vi "Channel to Multiplexer.vi"(9 "Polarity (F: Negative, T: Positive)":bool=TRUE, 11 "Multiplexer":T1) -> (1 "ext. Voltmeter":T2=enum."Short AC Sampler", 2 "Nulldetector":T2=enum."Short AC Sampler", 3 "Channel":T2=enum."Short AC Sampler")   [LabVIEW 2019, in "ACSVcontrol-driver.lvlib"]
doc: "Returns setting of multiplexer for selected polarity and channel. Does not set any devices, this is only to simplify setting of multiplexer.\n\nOutput \"Channel\" is used for setup JVS-nulldetector-DUT.\nOutput \"Nulldetector\" is used for direct measurement of DUT using nulldetector.\nOutput \"ext. Voltmeter\" is used for direct measurement of DUT using external voltmeter."
uses:
  ACSVcontrol-driver.lvlib
  Type Definitions/Multiplexer.ctl
  Type Definitions/Measurement Channel.ctl
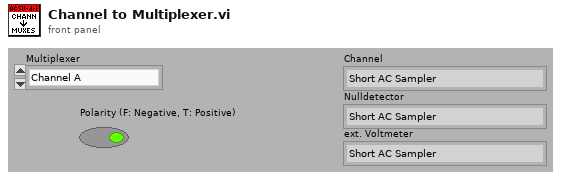
[diagram p1: front panel]
types:
  T1 = typedef "ACSVcontrol-driver.lvlib/Measurement Channel.ctl" = enum16{"Channel A", "Channel B", "Channel C"}
  T2 = typedef "ACSVcontrol-driver.lvlib/Multiplexer.ctl" = enum16{"Short DC Nano / Voltmeter", "Short AC Sampler", "Short Switch DC (JVS->Nano)", "Short Switch AC (JVS->Digit)", "JVS-Voltmeter", "Channel A positive", "Channel A negative", "Channel B positive", "Channel B negative", "Channel C positive", "Channel C negative", "Nulldetector-Channel A+", "Nulldetector-Channel A-", "Nulldetector-Channel B+", "Nulldetector-Channel B-", "Nulldetector-Channel C+", "Nulldetector-Channel C-", "ext.Voltmeter-Channel A+", "ext.Voltmeter-Channel A-", "ext.Voltmeter-Channel B+", "ext.Voltmeter-Channel B-", "ext.Voltmeter-Channel C+", "ext.Voltmeter-Channel C-"}
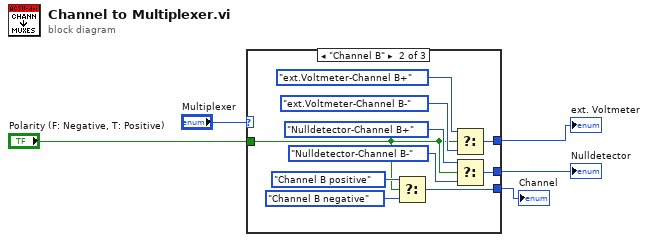
[diagram p0: block diagram]
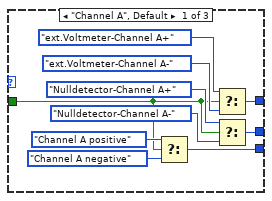
[diagram p2: hidden frame]
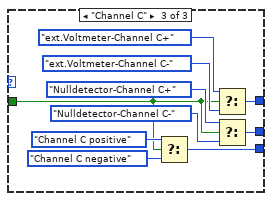
[diagram p3: hidden frame]
diagram:
  n1 = case shown="\"Channel B\"" "Multiplexer" {
    tunnel: "Polarity (F: Negative, T: Positive)" -> [w9 w19 w29]
    tunnel: [w8 w18 w28] -> w4
    tunnel: [w7 w17 w27] -> w3
    tunnel: [w6 w16 w26] -> w2
    frame "Channel A", Default {
      n2 = Select(t=Multiplexer."Channel A positive" ("Multiplexer"), s=w9, f=Multiplexer."Channel A negative" ("Multiplexer")) -> (s? t:f=w8:T2)
      n3 = Select(t=Multiplexer."ext.Voltmeter-Channel A+" ("Multiplexer"), s=w9, f=Multiplexer."ext.Voltmeter-Channel A-" ("Multiplexer")) -> (s? t:f=w6:T2)
      n4 = Select(t=Multiplexer."Nulldetector-Channel A+" ("Multiplexer"), s=w9, f=Multiplexer."Nulldetector-Channel A-" ("Multiplexer")) -> (s? t:f=w7:T2)
    }
    frame "Channel B" {
      n5 = Select(t=Multiplexer."Channel B positive" ("Multiplexer"), s=w19, f=Multiplexer."Channel B negative" ("Multiplexer")) -> (s? t:f=w18:T2)
      n6 = Select(t=Multiplexer."ext.Voltmeter-Channel B+" ("Multiplexer"), s=w19, f=Multiplexer."ext.Voltmeter-Channel B-" ("Multiplexer")) -> (s? t:f=w16:T2)
      n7 = Select(t=Multiplexer."Nulldetector-Channel B+" ("Multiplexer"), s=w19, f=Multiplexer."Nulldetector-Channel B-" ("Multiplexer")) -> (s? t:f=w17:T2)
    }
    frame "Channel C" {
      n8 = Select(t=Multiplexer."Channel C positive" ("Multiplexer"), s=w29, f=Multiplexer."Channel C negative" ("Multiplexer")) -> (s? t:f=w28:T2)
      n9 = Select(t=Multiplexer."ext.Voltmeter-Channel C+" ("Multiplexer"), s=w29, f=Multiplexer."ext.Voltmeter-Channel C-" ("Multiplexer")) -> (s? t:f=w26:T2)
      n10 = Select(t=Multiplexer."Nulldetector-Channel C+" ("Multiplexer"), s=w29, f=Multiplexer."Nulldetector-Channel C-" ("Multiplexer")) -> (s? t:f=w27:T2)
    }
  }
  "Channel" <- w4
  "Nulldetector" <- w3
  "ext. Voltmeter" <- w2
